vi "RD Digital Out Trigger Source Set.vi"(8 "error in (no error)":errorcluster caption="错误输入（无错误）", 10 "trigsrc":u8, 11 "handle":u64) -> (0 "error out":errorcluster caption="错误输出", 2 "function return":i32, 3 "handle out":u64)   [LabVIEW 2018, in "InstrumentsPlayground.lvlib"]
doc: "CLIFFAPI int CliffDigitalOutTriggerSourceSet(FT_HANDLE handle, CLIFFTRIGSRC trigsrc);\ntrigrs:\nNone = 0;\nDetectorAnalogInCH1 = 1;\nDetectorAnalogInCH2 = 2;\nAnalogOut1 = 3;\nAnalogOut2 = 4;\nDetectorDigitalIn = 5;\nDigitalOut = 6;\nManule = 7;\nExternal1 = 8;\nExternal2 = 9;\nDigitalIn =10;"
uses:
  InstrumentsPlayground.lvlib
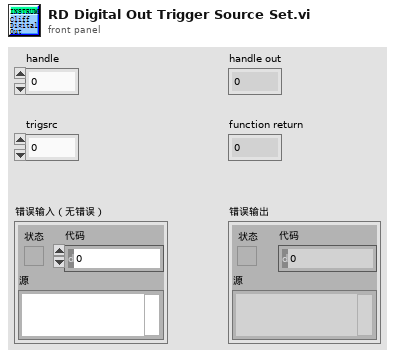
[diagram p1: front panel]
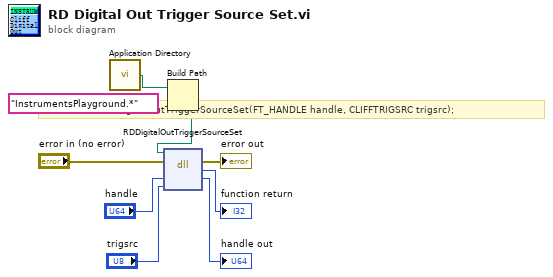
[diagram p0: block diagram]
diagram:
  # "CLIFFAPI int CliffDigitalOutTriggerSourceSet(FT_HANDLE handle, CLIFFTRIGSRC trigsrc);"
  n1 = call <vilib>:"Application Directory.vi"() -> ("Application Directory"=w2:path)
  n2 = Build Path(base path=w2, name or relative path="InstrumentsPlayground.*" ("名称或相对路径")) -> (appended path=w1:path)
  n3 = dll-call lib="E:/work/YZCourse_Xtext/Cliff/API/LabVIEW lib/InstrumentsPlayground.*" fn="RDDigitalOutTriggerSourceSet"(path in=w1, error in="error in (no error)", "handle"="handle", "trigsrc"="trigsrc") -> (error out=→"error out":errorcluster, "返回类型"=→"function return":i32, "handle"=→"handle out":u64)  [unwired: 2 in, 1 out]
